vi "write pair information.vi"(8 "error in":errorcluster, 10 "pair info":T1, 11 "UDP Broadcast Editor Node in":refnum<class "TEC editor node.lvclass">) -> (0 "error out":errorcluster, 3 "UDP Broadcast Editor Node out":refnum<class "TEC editor node.lvclass">)   [LabVIEW 2013, in "TEC editor node.lvclass"]
uses:
  TEC editor node.lvclass
  pair information.ctl
  pair type.ctl
  TEC editor node.lvclass/TEC editor node.ctl
  <vilib>/NI/Tag Bus Module Framework/root configuration/TBM configuration.lvclass
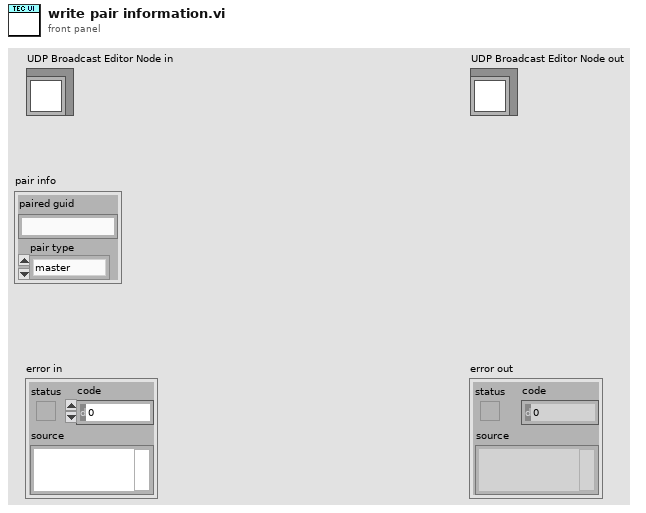
[diagram p1: front panel]
types:
  T1 = typedef "TEC editor node.lvclass/pair information.ctl" = cluster{"paired guid":string, "pair type":T2}
  T2 = typedef "TEC editor node.lvclass/pair type.ctl" = enum16{"master", "slave"}
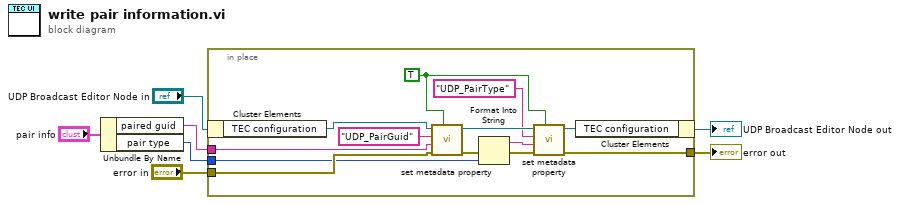
[diagram p0: block diagram]
diagram:
  n1 = Unbundle By Name("pair info") -> ("paired guid"=w2:string, "pair type"=w1:T2)
  n2 = in-place {
    in-place-border: "error in" -> [w17]
    in-place-border: [w16] -> w4
    in-place-border: w2 -> [w11]
    in-place-border: w1 -> [w8]
    w12 = TRUE ("overwrite?")
    n3 = in-place-cluster #1("UDP Broadcast Editor Node in") -> ("TEC configuration"=w20:refnum<class "TEC configuration.lvclass">)
    n4 = call <vilib>:"set metadata property.vi"("overwrite?"=w12, "error in"=w17, "value"=w11, "key"="UDP_PairGuid", "configuration in"=w20) -> ("error out"=w15:errorcluster, "configuration out"=w19:refnum<class "TEC configuration.lvclass">)  [unwired: 5 in]
    n5 = Format Into String(error in=w15, w8) -> (resulting string=w9:string, error out=w10:errorcluster)  [unwired: 2 in]
    n6 = call <vilib>:"set metadata property.vi"("overwrite?"=w12, "error in"=w10, "value"=w9, "key"="UDP_PairType", "configuration in"=w19) -> ("error out"=w16:errorcluster, "configuration out"=w18:refnum<class "TEC configuration.lvclass">)  [unwired: 5 in]
    n7 = in-place-cluster #1("TEC configuration"=w18) -> (→"UDP Broadcast Editor Node out":refnum<class "TEC editor node.lvclass">)
  }
  "error out" <- w4
